vi "HEWH Read Power OhioSemitronics.vi"(0 "VISA resource name":refnum<visa-resource-name>="MW100", 2 "Semiphore":T1, 11 "error in (no error)":errorcluster) -> (3 "PowerClass":T3={"Off"=FALSE, "On"=TRUE, "Fans"=FALSE, "Compressor"=FALSE, "Heat Elem."=TRUE, "Fault-OverPwr"=FALSE}, 4 "VISA resource name out":refnum<visa-resource-name>="MW100", 6 "PowerData":T2={"Voltage"=240.0, "Current"=0.017575, "Power"=4.218, "WattHours"=19682.0}, 15 "error out":errorcluster)   [LabVIEW 2012]
uses:
  PowerClassification.ctl
  PowerData.ctl
  ChannelSettings.ctl
panel:
  out "CycleCount":dbl
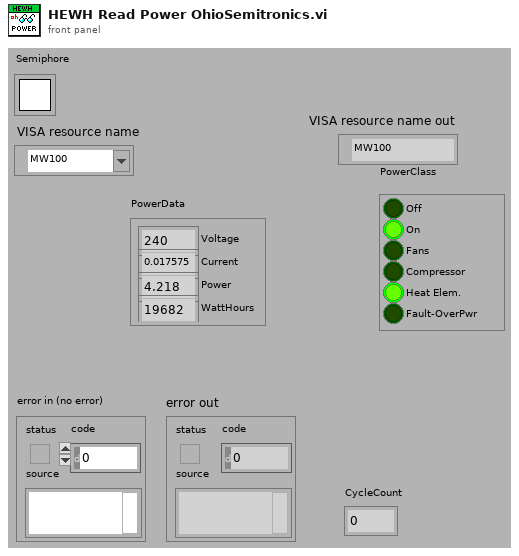
[diagram p1: front panel]
types:
  T1 = typedef "Semaphore RefNum" = refnum<k1>
  T2 = typedef "PowerData.ctl" = cluster{"Voltage":dbl, "Current":dbl, "Power":dbl, "WattHours":dbl}
  T3 = typedef "PowerClassification.ctl" = cluster{"Off":bool, "On":bool, "Fans":bool, "Compressor":bool, "Heat Elem.":bool, "Fault-OverPwr":bool}
  T4 = typedef "ChannelSettings.ctl" = u32
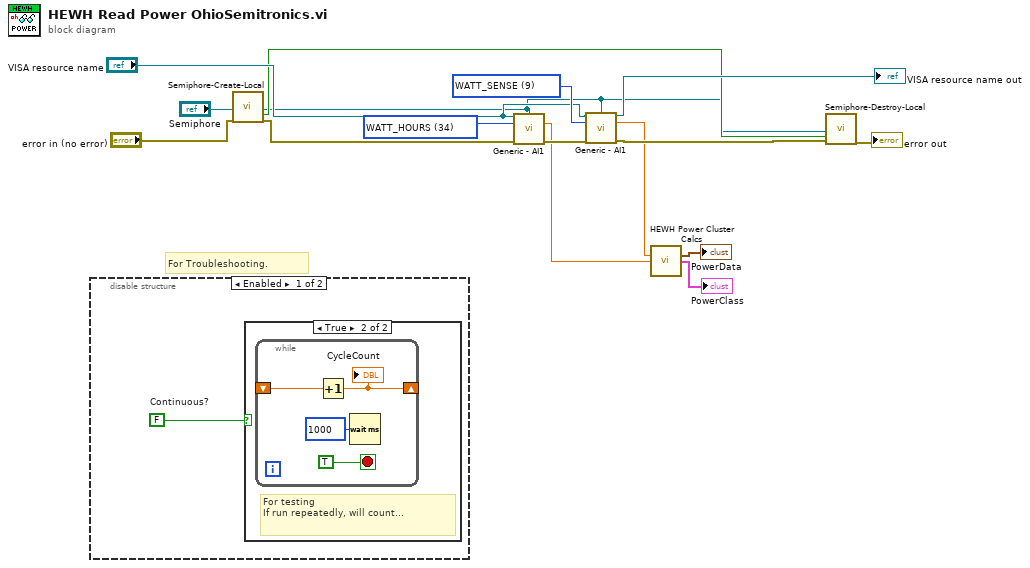
[diagram p0: block diagram]
diagram:
  w11 = T4 9 items=["4-20_OUT", "Pres_HI1", "Pres_HI2", "Pres_LOW", "Pres_PIN", "HEATER_TOP", "HEATER_BOT", "T_Shell", "FLOWMETER", "WATT_SENSE", "WH_TICK", "Tc_1", "Tc_2", "Tc_3", "Tc_4", "Tc_5", "Tc_6", "Tc_down", "T_Shell_2", "T_Shell_3", "T_Shell_4", "RTD_IN", "RTD_OUT", "RTD_AMB", "INTF_TEMPFLO", "INTF_READY", "INTF_START", "INTF_STOP", "DRM_LOW", "DRM_HIGH", "PWR_MAIN", "VLV_DUMP", "VLV_OUT", "VLV_IN", "WATT_HOURS", "FLOW(SAMPLE)", "GALLONS", "FLOW(GPM)"] ("Channel_Enum")
  w13 = T4 34 items=["4-20_OUT", "Pres_HI1", "Pres_HI2", "Pres_LOW", "Pres_PIN", "HEATER_TOP", "HEATER_BOT", "T_Shell", "FLOWMETER", "WATT_SENSE", "WH_TICK", "Tc_1", "Tc_2", "Tc_3", "Tc_4", "Tc_5", "Tc_6", "Tc_down", "T_Shell_2", "T_Shell_3", "T_Shell_4", "RTD_IN", "RTD_OUT", "RTD_AMB", "INTF_TEMPFLO", "INTF_READY", "INTF_START", "INTF_STOP", "DRM_LOW", "DRM_HIGH", "PWR_MAIN", "VLV_DUMP", "VLV_OUT", "VLV_IN", "WATT_HOURS", "FLOW(SAMPLE)", "GALLONS", "FLOW(GPM)"] ("Channel_Enum")
  # "For Troubleshooting."
  n1 = disable-structure shown="Enabled" {
    frame Enabled {
      w17 = FALSE  # Continuous?
      n2 = case shown="True" w17 {
        frame False {
        }
        frame True {
          # "For testing\nIf run repeatedly, will count..."
          n3 = while {
            shift-right: [w20] -> _
            shift-left: _ -> [w19]
            stop <- TRUE stop-if-true
            n4 = Increment(x=w19) -> (x+1=w20:dbl)
            "CycleCount" <- w20
            n5 = Wait (ms)(milliseconds to wait=u32 1000) -> ()  [unwired: 1 out]
          }
        }
      }
    }
    frame Disabled {
    }
  }
  n6 = call "Semiphore-Create-Local.vi"("Semiphore"="Semiphore", "error in (no error)"="error in (no error)") -> ("semaphore"=w5:T1, "Local?"=w8:bool, "error out"=w14:errorcluster)  [unwired: 15 in]
  n7 = call "Generic - AI1.vi"("MW100"="VISA resource name", "Semiphore"=w5, "Channel_Enum"=w13, "Error In"=w14) -> ("Value"=w1:dbl, "Error Out"=w12:errorcluster)  [unwired: 9 in, 1 out]
  n8 = call "Generic - AI1.vi"("MW100"="VISA resource name", "Semiphore"=w5, "Channel_Enum"=w11, "Error In"=w12) -> ("dup VISA session"=→"VISA resource name out":refnum<visa-resource-name>, "Value"=w2:dbl, "Error Out"=w7:errorcluster)  [unwired: 9 in]
  n9 = call "HEWH Power Cluster Calcs.vi"("Watts"=w2, "WattHours"=w1) -> ("PowerData"=→"PowerData":T2, "PowerClass"=→"PowerClass":T3)  [unwired: 12 in]
  n10 = call "Semiphore-Destroy-Local.vi"("Semiphore"=w5, "Local?"=w8, "error in (no error)"=w7) -> ("error out"=→"error out":errorcluster)  [unwired: 16 in]
